vi "Part 2.vi"(11 "Input":string) -> (3 "Output":i64)   [LabVIEW 2021]
panel:
  out "Player 2 Wins":i64
  out "Player 1 Wins":i64
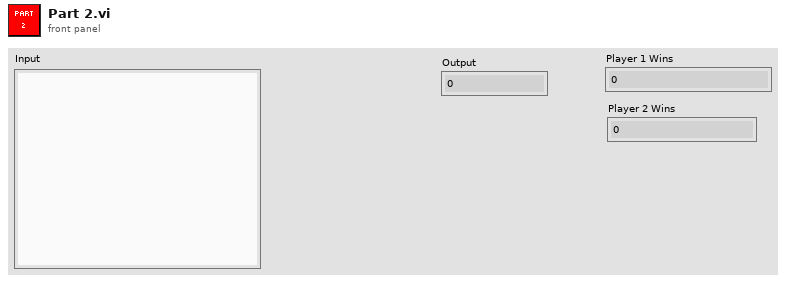
[diagram p1: front panel]
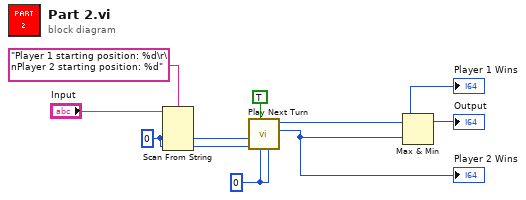
[diagram p0: block diagram]
diagram:
  w2 = i64 0 ("Player 1 Wins")
  w8 = i64 0 ("default value 1")
  n1 = Scan From String(format string="Player 1 starting position: %d\r\nPlayer 2 starting position: %d", input string="Input", default 1=w8, default 2=w8) -> (output 1=w3:i64, output 2=w1:i64)  [unwired: 2 in, 3 out]
  n2 = call "Play Next Turn.vi"("Player 2 Score"=w2, "Player 1 Score"=w2, "Player 1 Turn?"=TRUE, "Player 2 Position"=w1, "Player 1 Position"=w3) -> ("Player 2 Wins Out"=w5:i64, "Player 1 Wins Out"=w6:i64)  [unwired: 5 in]
  "Player 1 Wins" <- w6
  "Player 2 Wins" <- w5
  n3 = Max & Min(x=w6, y=w5) -> (max(x,y)=→"Output":i64)  [unwired: 1 out]
